vi "F PDF.vi"(9 "k2":i32=1, 10 "k1":i32=1, 11 "x":dbl=0.5) -> (0 "error":i32, 3 "pdf(x)":dbl=0.30010543871903544)   [LabVIEW 2010, in "NI_Gmath.lvlib"]
doc: "Computes the continuous probability density function (PDF) of various distributions. You must manually select the polymorphic instance to use."
uses:
  NI_Gmath.lvlib
  st_error_code.ctl
panel:
  # "F PDF"
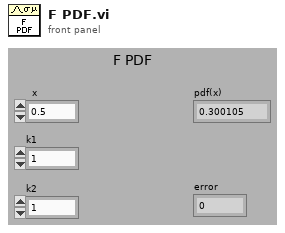
[diagram p1: front panel]
types:
  T1 = typedef "NI_Gmath.lvlib/st_error_code.ctl" = i32
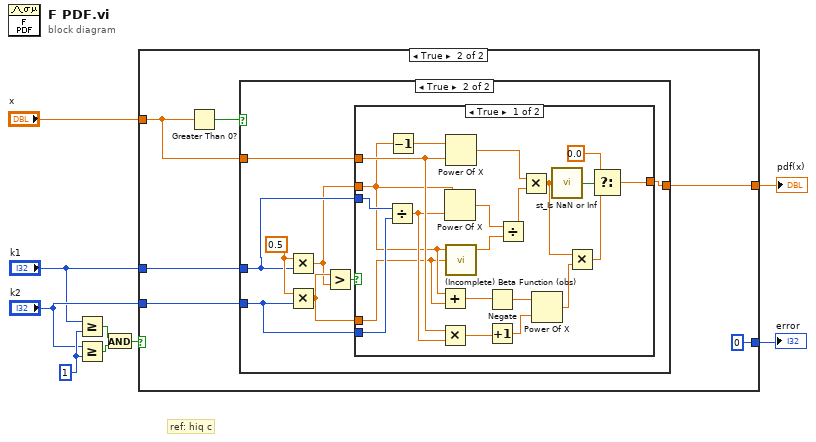
[diagram p0: block diagram]
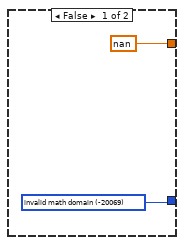
[diagram p2: hidden frame]
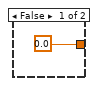
[diagram p3: hidden frame]
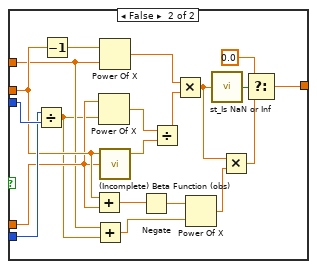
[diagram p4: hidden frame]
diagram:
  w3 = 1 ("y")
  # "ref: hiq c"
  n1 = Greater Or Equal?(x="k1", y=w3) -> (x >= y?=w4:bool)
  n2 = Greater Or Equal?(x="k2", y=w3) -> (x >= y?=w5:bool)
  n3 = And(x=w4, y=w5) -> (x .and. y?=w6:bool)
  n4 = case shown="True" w6 {
    tunnel: "k2" -> [_ w14]
    tunnel: [w10 0 ("invalid math domain")] -> w9
    tunnel: [nan w16] -> w8
    tunnel: "x" -> [_ w13]
    tunnel: "k1" -> [_ w15]
    frame False {
      w10 = T1 -20069 items=["invalid math domain"=-20069, "Fourier interpolation size m >= n"=-20070, "empty array"=-20003] ("stat interp error code")
    }
    frame True {
      n5 = Greater Than 0?(x=w13) -> (x > 0?=w12:bool)
      n6 = case shown="True" w12 {
        tunnel: [0.0 w19] -> w16
        tunnel: w13 -> [_ w20]
        tunnel: w15 -> [_ w22]
        tunnel: w14 -> [_ w24]
        frame False {
        }
        frame True {
          w26 = 0.5 ("x")
          n7 = Multiply(x=w26, y=w22) -> (x*y=w21:dbl)
          n8 = Multiply(x=w26, y=w24) -> (x*y=w23:dbl)
          n9 = Greater?(x=w23, y=w21) -> (0:w25:bool)
          n10 = case shown="True" w25 {
            tunnel: w24 -> [w46 w66]
            tunnel: w23 -> [w34 w52]
            tunnel: w22 -> [w47 w67]
            tunnel: w21 -> [w35 w58]
            tunnel: w20 -> [w38 w50]
            tunnel: [w28 w53] -> w19
            frame True {
              n11 = Divide(x=w47, y=w46) -> (x/y=w37:dbl)
              n12 = Decrement(x=w35) -> (x-1=w43:dbl)
              n13 = Add(x=w35, y=w34) -> (x+y=w27:dbl)
              n14 = Multiply(x=w38, y=w37) -> (x*y=w36:dbl)
              n15 = Power Of X(1:w37, 2:w35) -> (0:w44:dbl)
              n16 = Power Of X(1:w38, 2:w43) -> (0:w41:dbl)
              n17 = call "(Incomplete) Beta Function (obs).vi"("y"=w34, "x"=w35) -> ("b(x, y, a)"=w45:dbl)  [unwired: 3 in]
              n18 = Negate(x=w27) -> (-x=w33:dbl)
              n19 = Increment(x=w36) -> (x+1=w30:dbl)
              n20 = Divide(x=w44, y=w45) -> (x/y=w42:dbl)
              n21 = Multiply(x=w41, y=w42) -> (x*y=w31:dbl)
              n22 = Power Of X(1:w30, 2:w33) -> (0:w32:dbl)
              n23 = call "st_Is NaN or Inf.vi"("x"=w31) -> ("isNaN(x) || isInf(x)"=w40:bool)  [unwired: 4 in]
              n24 = Multiply(x=w31, y=w32) -> (x*y=w29:dbl)
              n25 = Select(t=0.0, s=w40, f=w29) -> (s? t:f=w28:dbl)
            }
            frame False {
              n26 = Divide(x=w66, y=w67) -> (x/y=w49:dbl)
              n27 = Decrement(x=w58) -> (x-1=w63:dbl)
              n28 = Add(x=w58, y=w52) -> (x+y=w51:dbl)
              n29 = Add(x=w50, y=w49) -> (x+y=w48:dbl)
              n30 = Power Of X(1:w49, 2:w52) -> (0:w64:dbl)
              n31 = Power Of X(1:w50, 2:w63) -> (0:w61:dbl)
              n32 = call "(Incomplete) Beta Function (obs).vi"("y"=w52, "x"=w58) -> ("b(x, y, a)"=w65:dbl)  [unwired: 3 in]
              n33 = Negate(x=w51) -> (-x=w57:dbl)
              n34 = Divide(x=w64, y=w65) -> (x/y=w62:dbl)
              n35 = Multiply(x=w61, y=w62) -> (x*y=w55:dbl)
              n36 = Power Of X(1:w48, 2:w57) -> (0:w56:dbl)
              n37 = call "st_Is NaN or Inf.vi"("x"=w55) -> ("isNaN(x) || isInf(x)"=w60:bool)  [unwired: 4 in]
              n38 = Multiply(x=w55, y=w56) -> (x*y=w54:dbl)
              n39 = Select(t=0.0, s=w60, f=w54) -> (s? t:f=w53:dbl)
            }
          }
        }
      }
    }
  }
  "pdf(x)" <- w8
  "error" <- w9
